vi "Example - Simple.vi"() -> ()   [LabVIEW 2017]
uses:
  AI_class/AI.lvclass
panel:
  out "AI Signal is Zero":bool[](array[boolean])
  out "AI Signal Chart":dbl[][](graph)
  out "AI Chanel Standard Deviations":dbl[](array[numeric])
  out "AI Channel Averages":dbl[](array[numeric])
  out "AI Readings":dbl[][](array[numeric])
  in  "Quit Program":bool
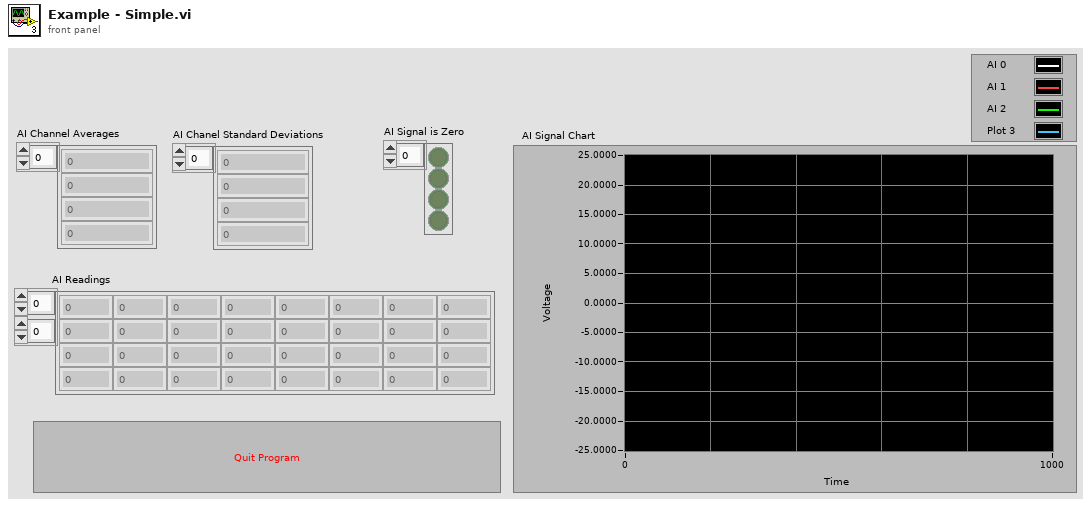
[diagram p1: front panel]
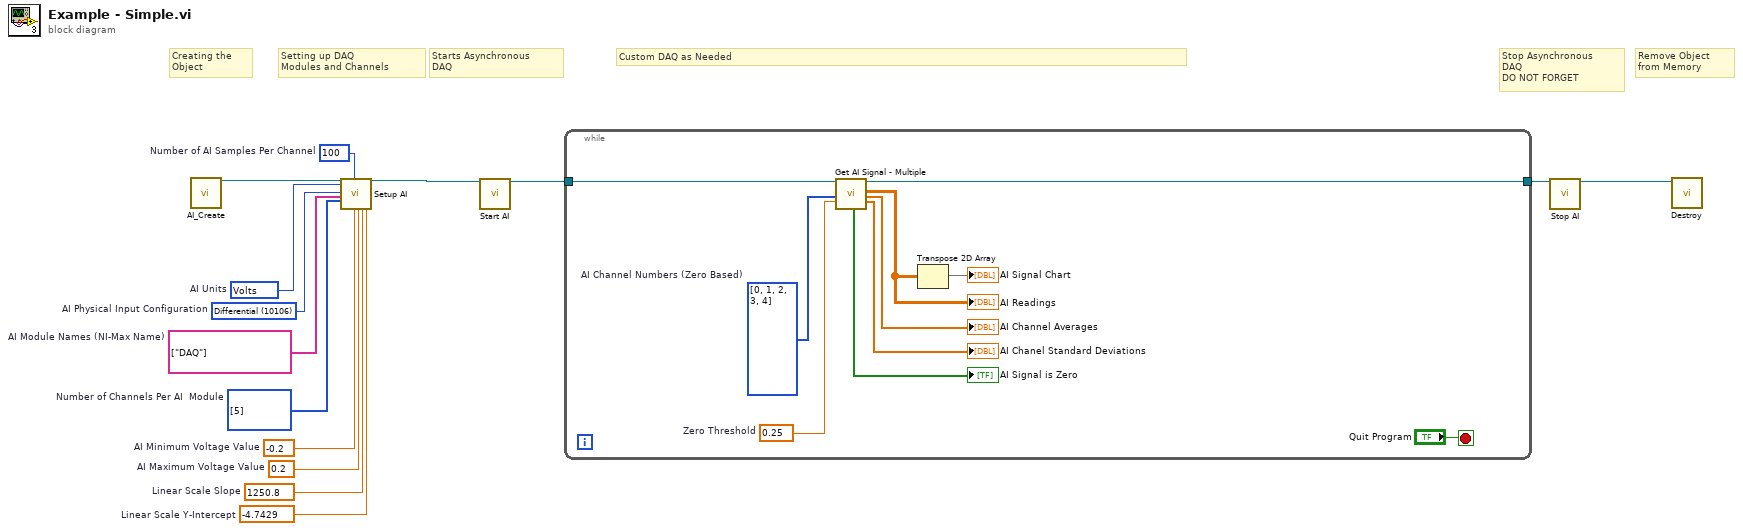
[diagram p0: block diagram]
diagram:
  w1 = -4.7429  # Linear Scale Y-Intercept
  w2 = 1250.8  # Linear Scale Slope
  w3 = 10348 items=["Volts"=10348, "From Custom Scale"=10065]  # AI Units
  w4 = 0.2  # AI Maximum Voltage Value
  w5 = -0.2  # AI Minimum Voltage Value
  w6 = 100  # Number of AI Samples Per Channel
  w7 = 10106 items=["Default"=-1, "RSE"=10083, "NRSE"=10078, "Differential"=10106, "Pseudodifferential"=12529]  # AI Physical Input Configuration
  w8 = string[] ["DAQ"]  # AI Module Names (NI-Max Name)
  w9 = i32[] [5]  # Number of Channels Per AI  Module
  # "Creating the\nObject"
  # "Setting up DAQ\nModules and Channels"
  # "Custom DAQ as Needed"
  # "Remove Object\nfrom Memory"
  # "Stop Asynchronous\nDAQ\nDO NOT FORGET"
  # "Starts Asynchronous\nDAQ"
  n1 = call "AI_Create.vi"() -> ("reference out"=w14:refnum<class "AI.lvclass">)  [unwired: 18 in, 1 out]
  n2 = call-dynamic "Setup AI.vi"("reference in"=w14, "AI Units"=w3, "AI Physical Input Configuration"=w7, "AI Module Names (NI-Max Name)"=w8, "Number of Channels Per AI  Module"=w9, "Number of AI Samples Per Channel"=w6, "AI Minimum Voltage Value"=w5, "AI Maximum Voltage Value"=w4, "Linear Scale Slope"=w2, "Linear Scale Y-Intercept"=w1) -> ("reference out"=w13:refnum<class "AI.lvclass">)  [unwired: 16 in, 1 out]
  n3 = call-dynamic "Start AI.vi"("reference in"=w13) -> ("reference out"=w11:refnum<class "AI.lvclass">)  [unwired: 17 in, 1 out]
  n4 = while {
    tunnel: w11 -> [w23]
    tunnel: [w15] -> w10
    stop <- "Quit Program" stop-if-true
    w16 = 0.25  # Zero Threshold
    w19 = i32[] [0, 1, 2, 3, 4]  # AI Channel Numbers (Zero Based)
    n5 = call-dynamic "Get AI Signal - Multiple.vi"("reference in"=w23, "AI Channel Numbers (Zero Based)"=w19, "Zero Threshold"=w16) -> ("AI Channel Signal is Zero"=→"AI Signal is Zero":bool[], "reference out"=w15:refnum<class "AI.lvclass">, "AI Channel Readings"=w18:dbl[][], "AI Channel Average"=→"AI Channel Averages":dbl[], "AI Channel Standard Deviation"=→"AI Chanel Standard Deviations":dbl[])  [unwired: 11 in, 1 out]
    "AI Readings" <- w18
    n6 = Transpose 2D Array(2D array=w18) -> (transposed array=→"AI Signal Chart":dbl[][])
  }
  n7 = call-dynamic "Stop AI.vi"("reference in"=w10) -> ("reference out"=w12:refnum<class "AI.lvclass">)  [unwired: 17 in, 1 out]
  n8 = call-dynamic "Destroy.vi"("reference in"=w12) -> ()  [unwired: 17 in, 2 out]
